vi "ExportPacket.vi"(6 "ExportType":T1, 9 "Comment":string, 10 "GyroData":waveform(dbl)[](graph), 11 "AccelData":waveform(dbl)[](graph)) -> (0 "ErrorOut":errorcluster, 1 "Exported?":bool)   [LabVIEW 2016]
uses:
  ExportPacket/ExportType.ctl
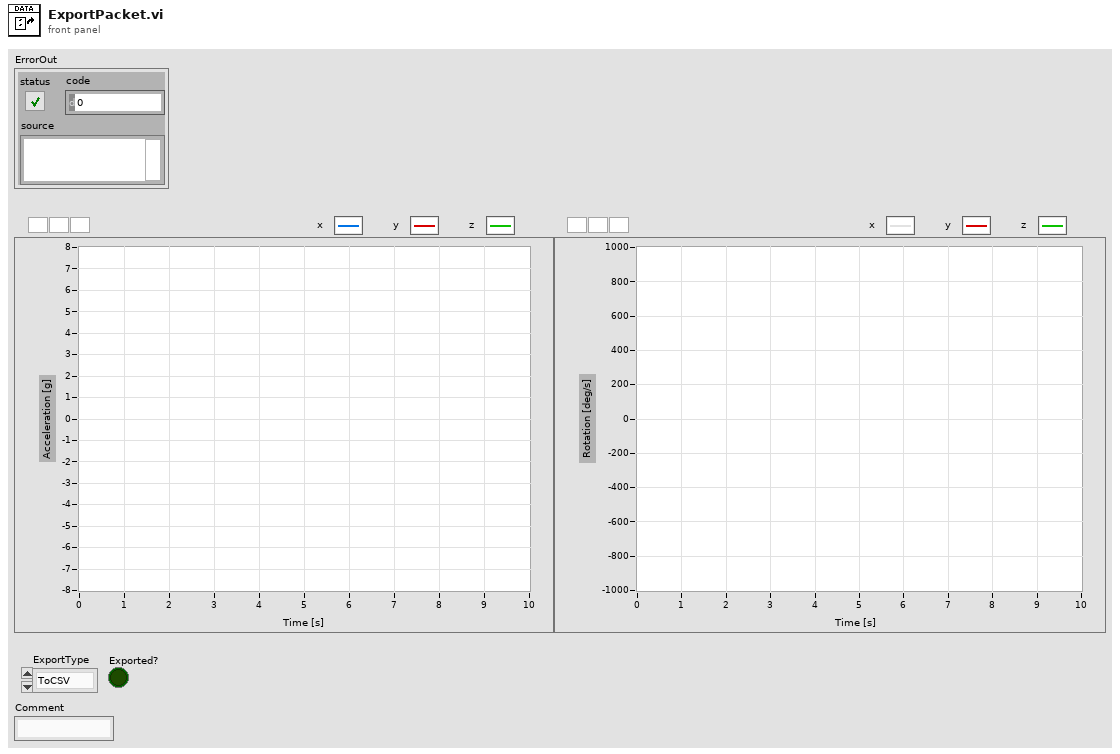
[diagram p1: front panel]
types:
  T1 = typedef "ExportType.ctl" = enum16{"ToCSV", "ToJSON"}
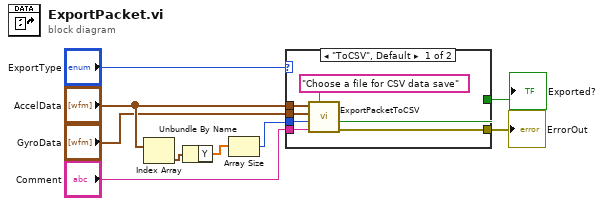
[diagram p0: block diagram]
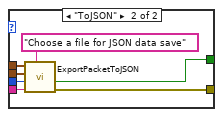
[diagram p2: hidden frame]
diagram:
  n1 = Index Array(array="AccelData") -> (element=w9:waveform(dbl))  [unwired: 1 in]
  n2 = Unbundle By Name(w9) -> ("Y"=w8:dbl[])
  n3 = Array Size(array=w8) -> (size(s)=w7:i32)
  n4 = case shown="\"ToCSV\", Default" "ExportType" {
    tunnel: w7 -> [w16 w22]
    tunnel: "AccelData" -> [w15 w23]
    tunnel: "GyroData" -> [w14 w20]
    tunnel: [w13 w21] -> w4
    tunnel: [w12 w19] -> w2
    tunnel: "Comment" -> [w11 w18]
    frame "ToCSV", Default {
      n5 = call "ExportPacketToCSV.vi"("Prompt"="Choose a file for CSV data save", "Comment"=w11, "NumerOfSamplesForAxis"=w16, "GyroData"=w14, "AccelData"=w15) -> ("ErrorOut"=w13:errorcluster, "Exported?"=w12:bool)  [unwired: 5 in]
    }
    frame "ToJSON" {
      n6 = call "ExportPacketToJSON.vi"("Prompt"="Choose a file for JSON data save", "Comment"=w18, "NumerOfSamplesForAxis"=w22, "GyroData"=w20, "AccelData"=w23) -> ("ErrorOut"=w21:errorcluster, "Exported?"=w19:bool)  [unwired: 5 in]
    }
  }
  "ErrorOut" <- w4
  "Exported?" <- w2
